vi "labviewtest1.vi"() -> ()   [LabVIEW 2017]
uses:
  <vilib>/LabVIEW Interface for Arduino/Type Defs/Connection Type.ctl
  <vilib>/LabVIEW Interface for Arduino/Type Defs/Board Type.ctl
  <vilib>/LabVIEW Interface for Arduino/Type Defs/Pin Mode.ctl
  <vilib>/LabVIEW Interface for Arduino/LabVIEW Interface for Arduino.lvlib
panel:
  in  "Boolean":bool
  out "error out":errorcluster
  in  "stop":bool
  in  "VISA resource":refnum<visa-resource-name>
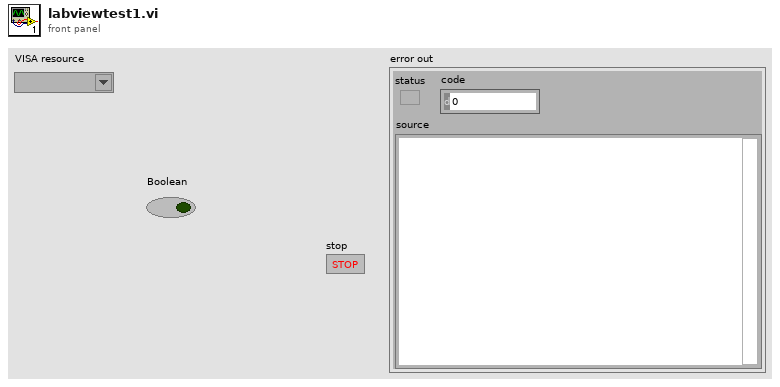
[diagram p1: front panel]
types:
  T1 = typedef "LabVIEW Interface for Arduino.lvlib/Pin Mode.ctl" = enum8{"Input", "Output"}
  T2 = typedef "LabVIEW Interface for Arduino.lvlib/Board Type.ctl" = enum16{"Uno", "Dimuelanove w/Atmega 328", "Mega 2560"}
  T3 = typedef "LabVIEW Interface for Arduino.lvlib/Connection Type.ctl" = enum8{"USB / Serial", "XBEE", "BlueSmirf (Bluetooth)"}
  T4 = typedef "LabVIEW Interface for Arduino.lvlib/Arduino Resource.ctl" = cluster{"VISA resource":refnum<visa-resource-name>, "Board Type":T2, "Connection Type":enum8{"USB / Serial"}, "Bytes Per Packet (15)":u8}
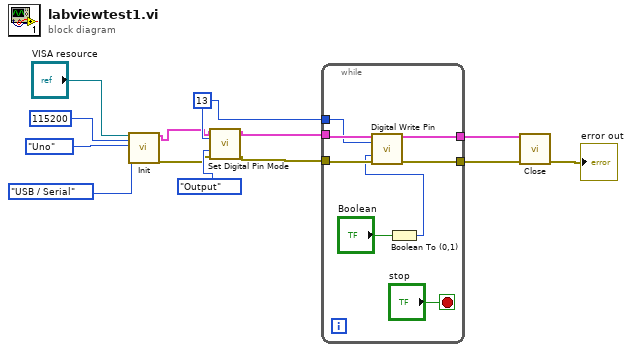
[diagram p0: block diagram]
diagram:
  w6 = u8 13 ("Digital I/O Pin")
  n1 = call <vilib>:"Init.vi"("VISA resource"="VISA resource", "Baud Rate (115200)"=u32 115200, "Board Type (Uno)"=Board_Type."Uno", "Connection Type (USB/Serial)"=Connection_Type."USB / Serial") -> ("Arduino Resource"=w1:T4, "error out"=w4:errorcluster)  [unwired: 14 in]
  n2 = call <vilib>:"Set Digital Pin Mode.vi"("Arduino Resource"=w1, "Digital I/O Pin"=w6, "Pin Mode (Input)"=Pin_Mode."Output", "error in"=w4) -> ("Arduino Resource"=w2:T4, "error out"=w3:errorcluster)  [unwired: 10 in]
  n3 = while {
    tunnel: w3 -> [w20]
    tunnel: w2 -> [w21]
    tunnel: w6 -> [w19]
    tunnel: [w18] -> w8
    tunnel: [w17] -> w9
    stop <- "stop" stop-if-true
    n4 = Boolean To (0,1)(Boolean="Boolean") -> (0, 1=w14:i16)
    n5 = call <vilib>:"Digital Write Pin.vi"("Arduino Resource"=w21, "Digital I/O Pin (0)"=w19, "Value (0)"=w14, "error in"=w20) -> ("Arduino Resource"=w18:T4, "error out"=w17:errorcluster)  [unwired: 10 in]
  }
  n6 = call <vilib>:"Close.vi"("Arduino Resource"=w8, "error in"=w9) -> ("error out"=→"error out":errorcluster)  [unwired: 13 in]
